vi "Synth Get Actual Frequency.vi"(11 "f-word":u32) -> (2 "Freq step":ext format="%_20p", 3 "Actual frequency, Hz":ext format="%_20p")   [LabVIEW 2016]
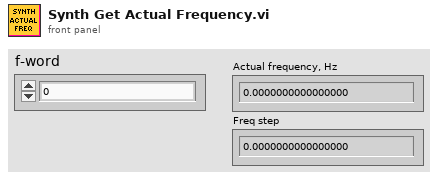
[diagram p1: front panel]
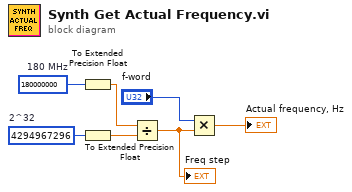
[diagram p0: block diagram]
diagram:
  w6 = u64 4294967296  # 2^32
  w7 = u64 180000000  # 180 MHz
  n1 = To Extended Precision Float(1:w7) -> (0:w5:ext)
  n2 = To Extended Precision Float(1:w6) -> (0:w4:ext)
  n3 = Divide(x=w5, y=w4) -> (x/y=w1:ext)
  "Freq step" <- w1
  n4 = Multiply(x="f-word", y=w1) -> (x*y=→"Actual frequency, Hz":ext)
